vi "DSF.Engine.BuilderManager.Set Builder States Pointer.vi"(10 "Builder States":refnum<class "DSF.Engine.Pointer.Status.Builder.State.lvclass">, 11 "Builder Manager in":refnum<class "DSF.Engine.BuilderManager.lvclass">) -> (3 "Builder Manager out":refnum<class "DSF.Engine.BuilderManager.lvclass">)   [LabVIEW 2016, in "DSF.Engine.lvlib" / "DSF.Engine.BuilderManager.lvclass"]
uses:
  DSF.Engine.BuilderManager.lvclass
  Pointer/DSF.Engine.Pointer.Status.Builder.State.lvclass
  DSF.Engine.BuilderManager.lvclass/DSF.Engine.BuilderManager.ctl
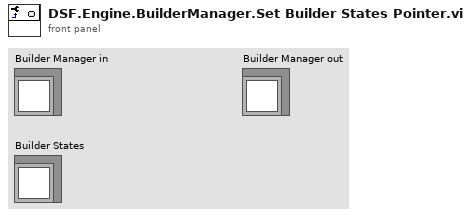
[diagram p1: front panel]
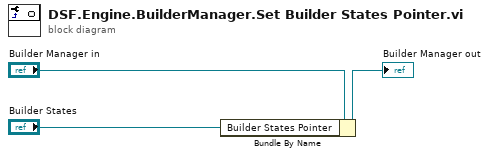
[diagram p0: block diagram]
diagram:
  n1 = Bundle By Name(cluster="Builder Manager in", "Builder States Pointer"="Builder States") -> (→"Builder Manager out":refnum<class "DSF.Engine.BuilderManager.lvclass">)
